vi "CustomData.vi"(5 "EndTime":timestamp, 7 "StartTime":timestamp, 8 "error in":errorcluster, 11 "CustomData":refnum<class "CustomData.lvclass">) -> (0 "error out":errorcluster, 3 "Passed":bool)   [LabVIEW 2020]
uses:
  <vilib>/Averna/ProligentResultProcessor/ProligentResultProcessor.lvlibp/Model/CustomData/CustomData.lvclass
  <vilib>/Averna/ProligentResultProcessor/ProligentResultProcessor.lvlibp/Model/CustomElement/SetValue.vi
  <vilib>/Averna/ProligentResultProcessor/ProligentResultProcessor.lvlibp/Model/CustomElement/GetValue.vi
  <vilib>/Averna/ProligentResultProcessor/ProligentResultProcessor.lvlibp/Model/CustomData/GetCustomElement.vi
  <vilib>/Averna/ProligentResultProcessor/ProligentResultProcessor.lvlibp/Model/CustomElement/CustomElement.lvclass
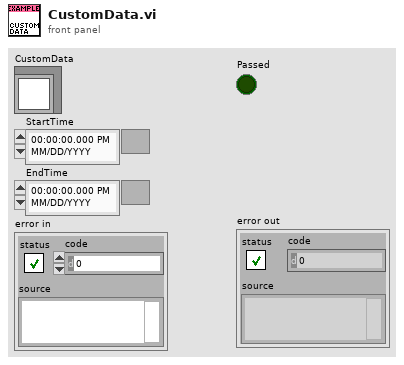
[diagram p1: front panel]
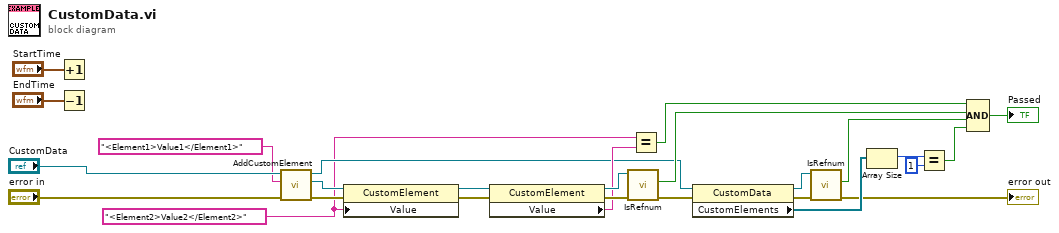
[diagram p0: block diagram]
diagram:
  w2 = "<Element2>Value2</Element2>"
  n1 = Increment(x="StartTime") -> ()  [unwired: 1 out]
  n2 = Decrement(x="EndTime") -> ()  [unwired: 1 out]
  n3 = call <vilib>:"AddCustomElement.vi"("error in"="error in", "Element"="<Element1>Value1</Element1>", "CustomData in"="CustomData") -> ("error out"=w12:errorcluster, "CustomElement"=w13:refnum<class "CustomElement.lvclass">, "CustomData out"=w3:refnum<class "CustomData.lvclass">)  [unwired: 6 in]
  n4 = property class="CustomElement"(reference=w13, error in=w12, "Value"=w2) -> (reference out=w10:refnum<class "CustomElement.lvclass">, error out=w11:errorcluster)
  n5 = property class="CustomElement"(reference=w10, error in=w11) -> (reference out=w8:refnum<class "CustomElement.lvclass">, error out=w9:errorcluster, "Value"=w7:string)
  n6 = call <vilib>:"IsRefnum.vi"("error in"=w9, "CustomElement in"=w8) -> ("error out"=w4:errorcluster, "IsRefnum"=w5:bool)  [unwired: 7 in, 1 out]
  n7 = Equal?(x=w2, y=w7) -> (x = y?=w6:bool)
  n8 = property class="CustomData"(reference=w3, error in=w4) -> (reference out=w18:refnum<class "CustomData.lvclass">, error out=w17:errorcluster, "CustomElements"=w16:refnum<class "CustomElement.lvclass">[])
  n9 = call <vilib>:"IsRefnum.vi"("error in"=w17, "CustomDataType in"=w18) -> ("error out"=→"error out":errorcluster, "IsRefnum"=w14:bool)  [unwired: 7 in, 1 out]
  n10 = Array Size(array=w16) -> (size(s)=w26:i32)
  n11 = Equal?(x=w26, y=1) -> (x = y?=w24:bool)
  n12 = Compound Arithmetic op=AND(w6, w5, w14, w24) -> (→"Passed":bool)
